vi "sweep.vi"(8 "Error in":errorcluster, 9 "Stop (Hz)":u32, 10 "Start (Hz)":u32, 11 "VISA name in":refnum<visa-resource-name>) -> (0 "Error out":errorcluster, 3 "VISA name out":refnum<visa-resource-name>)   [LabVIEW 2012]
panel:
  out "cmd terminate":string="\r\n"
  out "cmd echo":string="\r\n"
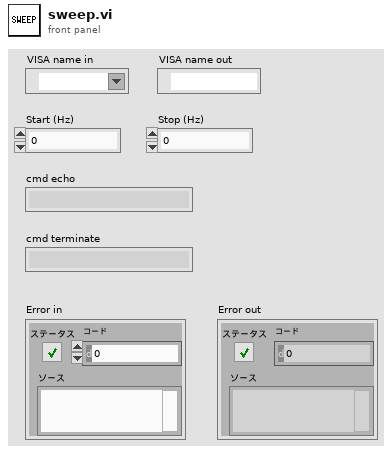
[diagram p1: front panel]
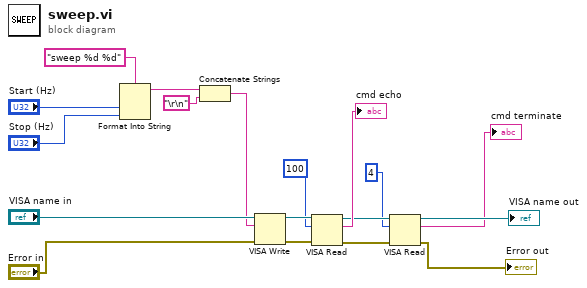
[diagram p0: block diagram]
diagram:
  n1 = Format Into String(format string="sweep %d %d" ("形式文字列"), "Start (Hz)", "Stop (Hz)") -> (resulting string=w10:string)  [unwired: 2 in, 1 out]
  n2 = Concatenate Strings(w10, "\r\n") -> (w8:string)
  n3 = VISA Write(VISA resource name="VISA name in", write buffer=w8, error in (no error)="Error in") -> (VISA resource name out=w17:refnum<visa-resource-name>, error out=w16:errorcluster)  [unwired: 1 out]
  n4 = VISA Read(VISA resource name=w17, byte count=u32 100 ("バイトカウント"), error in (no error)=w16) -> (VISA resource name out=w13:refnum<visa-resource-name>, read buffer=→"cmd echo":string, error out=w4:errorcluster)  [unwired: 1 out]
  n5 = VISA Read(VISA resource name=w13, byte count=u32 4 ("バイトカウント"), error in (no error)=w4) -> (VISA resource name out=→"VISA name out":refnum<visa-resource-name>, read buffer=→"cmd terminate":string, error out=→"Error out":errorcluster)  [unwired: 1 out]
